vi "QTab DEMO-Sub2.vi"() -> ()   [LabVIEW 2020]
panel:
  in  "Multicolumn Listbox":i32(listbox)
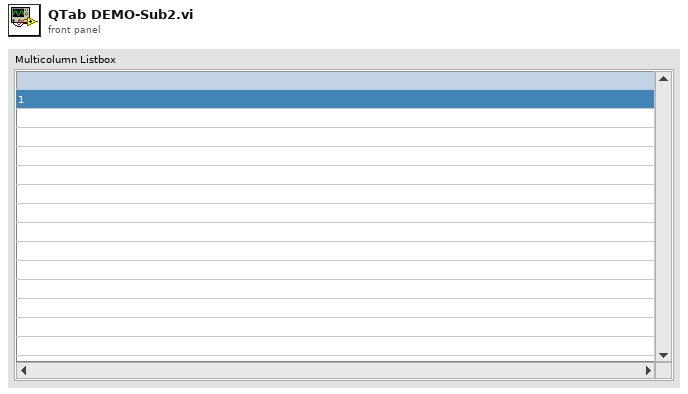
[diagram p1: front panel]
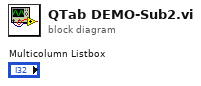
[diagram p0: block diagram]
diagram:
